vi "Funct img modulation core.vi"(8 "Pockels stay ON for at least this number of us after dwell time":dbl, 9 "Pockels turn ON at least this number of us before fill time completion":dbl, 11 "ROI setup":T1[](array[typedef]) {"ROI group ID" format="%#_6f"; "Laser Power (%)" format="%#_6f"; "Zoom" format="%#_6f"; "Frame Size" format="%#_6f"; "Number of lines" format="%#_6f"; "Composite ID" format="%#_6f"; "Angle (deg)" format="%#_6f"; "ROI Time (ns)" format="%#_6f"; "ROI ID" format="%#_6f"; "Pixels in ROI" format="%#_6f"; "ROI index" format="%#_6f"; "Z stop" format="%#_6f"; "Y stop" format="%#_6f"; "X stop" format="%#_6f"; "Z start" format="%#_6f"; "X start" format="%#_6f"; "Y start" format="%#_6f"}) -> (1 "AO card sampling interval (us)":dbl=1.0 format="%#_13g us", 2 "Fill time (us)":dbl=24.4 format="%#_g us", 3 "waveform out":waveform(dbl), 5 "ROI Dwell Time (us)":dbl)   [LabVIEW 2013]
uses:
  User Interface/Visualisation/Functional Imaging Viewer/Typedefs/ROI parameters data type.ctl
  Typedefs/Rounding type.ctl
  Global Variables/General Globals.vi
  Globals/gl_Pockels control globals.vi
  <vilib>/Waveform/WDTOps.llb/WDT Append Waveforms DBL.vi
panel:
  in  "Disable modulation":bool
  out "Pockels modulation signal":waveform(dbl)(graph)
  out "Remainder (us)":dbl
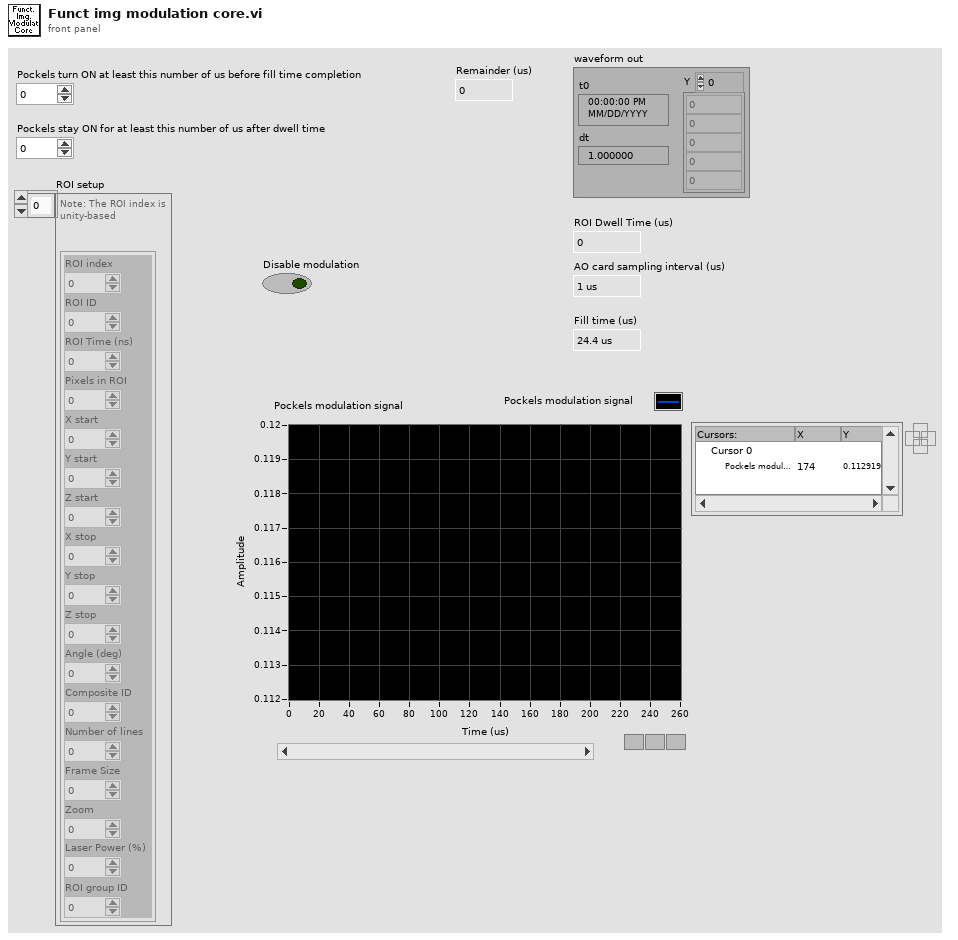
[diagram p1: front panel]
types:
  T1 = typedef "ROI parameters data type.ctl" = cluster{"ROI index":dbl, "ROI ID":dbl, "ROI Time (ns)":dbl, "Pixels in ROI":dbl, "X start":dbl, "Y start":dbl, "Z start":dbl, "X stop":dbl, "Y stop":dbl, "Z stop":dbl, "Angle (deg)":dbl, "Composite ID":dbl, "Number of lines":dbl, "Frame Size":dbl, "Zoom":dbl, "Laser Power (%)":dbl, "ROI group ID":dbl}
  T2 = typedef "Rounding type.ctl" = enum16{"No rounding", "Toward +Inf", "Toward -Inf"}
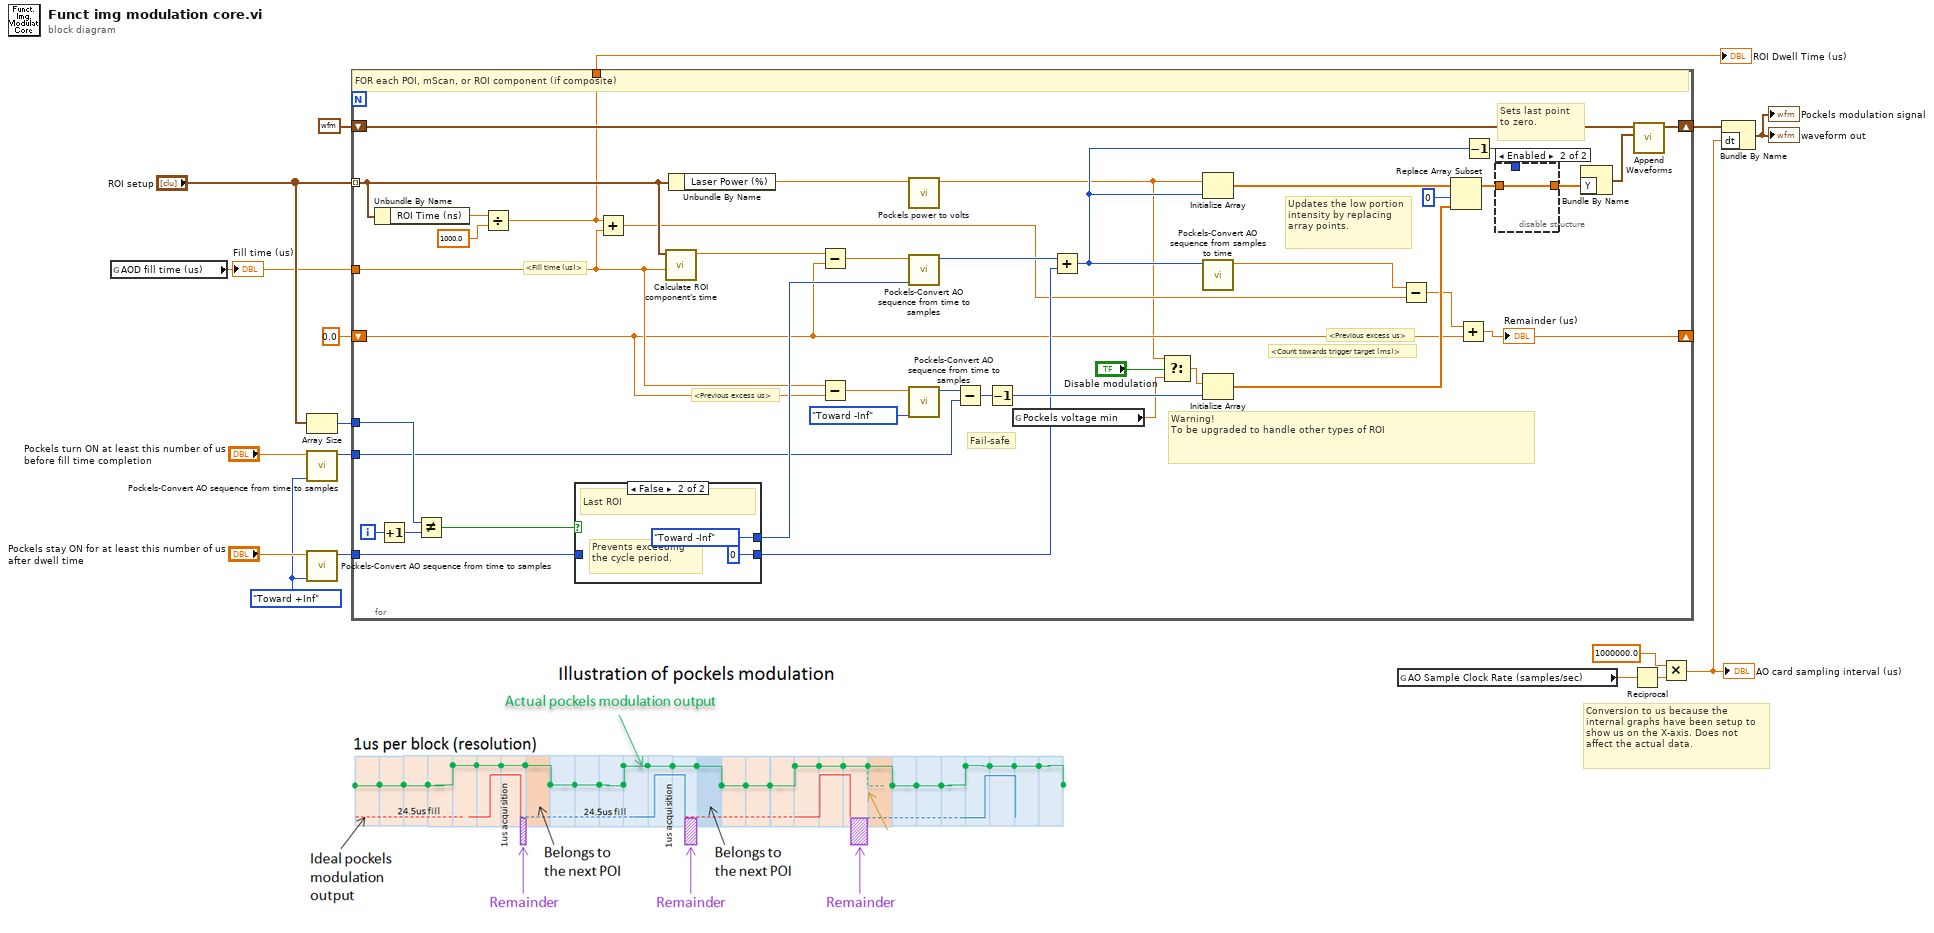
[diagram p0: block diagram]
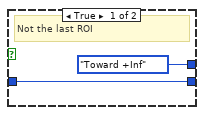
[diagram p2: hidden frame]
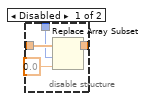
[diagram p3: hidden frame]
diagram:
  w4 = Rounding_type."Toward +Inf" ("Direction (+Inf)")
  # "Conversion to us because the internal graphs have been setup to show us on the X-axis. Does not affect the actual data."
  n1 = global read "General Globals.vi" "AOD fill time (us)"() -> (w8:dbl)
  "Fill time (us)" <- w8
  n2 = Array Size(array="ROI setup") -> (size(s)=w6:i32)
  n3 = call "Pockels-Convert AO sequence from time to samples.vi"("Direction (+Inf)"=w4, "Duration of AO sequence (us)"="Pockels turn ON at least this number of us before fill time completion") -> ("Number of samples in AO sequence"=w5:i32)  [unwired: 9 in]
  n4 = call "Pockels-Convert AO sequence from time to samples.vi"("Direction (+Inf)"=w4, "Duration of AO sequence (us)"="Pockels stay ON for at least this number of us after dwell time") -> ("Number of samples in AO sequence"=w3:i32)  [unwired: 9 in]
  n5 = for {
    tunnel: "ROI setup" -> [w50] mode=indexing
    shift-right: [w45] -> w13
    shift-left: waveform(dbl) {"t0"=timestamp(0 s since 1904-01-01), "dt"=0.0, "Y"=[]} ("waveform out") -> [w55]
    tunnel: w3 -> [w33]
    tunnel: w5 -> [w27]
    shift-right: [w19] -> _
    shift-left: 0.0 ("Count towards trigger target (us)") -> [w28]
    tunnel: w6 -> [w37]
    tunnel: [w35] -> w17
    tunnel: w8 -> [w29]
    i -> [w39]
    # "Updates the low portion intensity by replacing array points."
    # "<Previous excess us>"
    # "<Fill time (us)>"
    # "Warning!\nTo be upgraded to handle other types of ROI"
    # "<Previous excess us>"
    # "<Count towards trigger target (ms)>"
    # "Fail-safe"
    # "Sets last point to zero."
    # "FOR each POI, mScan, or ROI component (if composite)"
    n6 = Unbundle By Name(w50) -> ("ROI Time (ns)"=w36:dbl)
    n7 = Increment(x=w39) -> (x+1=w38:i32)
    n8 = Not Equal?(x=w37, y=w38) -> (x != y?=w24:bool)
    n9 = Divide(x=w36, y=1000.0) -> (x/y=w35:dbl)
    n10 = case shown="False" w24 {
      tunnel: [Rounding_type."Toward +Inf" ("Direction (+Inf)") Rounding_type."Toward -Inf" ("Direction (+Inf)")] -> w31
      tunnel: w33 -> [w60 _]
      tunnel: [w60 0 ("f")] -> w32
      frame True {
        # "Not the last ROI"
      }
      frame False {
        # "Prevents exceeding the cycle period."
        # "Last ROI"
      }
    }
    n11 = Add(x=w35, y=w29) -> (x+y=w26:dbl)
    n12 = call "Calculate ROI component's time.vi"("AOD fill time (us)"=w29, "Normalised ROI setup"=w50) -> ("ROI component's time (us)"=w48:dbl)  [unwired: 9 in]
    n13 = Unbundle By Name(w50) -> ("Laser Power (%)"=w58:dbl)
    n14 = Subtract(x=w48, y=w28) -> (x-y=w47:dbl)
    n15 = Subtract(x=w29, y=w28) -> (x-y=w46:dbl)
    n16 = call "Pockels power to volts.vi"("Pockels power (%)"=w58) -> ("Pockels control voltage (V)"=w21:dbl)  [unwired: 8 in, 2 out]
    n17 = call "Pockels-Convert AO sequence from time to samples.vi"("Direction (+Inf)"=w31, "Duration of AO sequence (us)"=w47) -> ("Number of samples in AO sequence"=w54:i32)  [unwired: 9 in]
    n18 = call "Pockels-Convert AO sequence from time to samples.vi"("Direction (+Inf)"=Rounding_type."Toward -Inf", "Duration of AO sequence (us)"=w46) -> ("Number of samples in AO sequence"=w53:i32)  [unwired: 9 in]
    n19 = Subtract(x=w53, y=w27) -> (x-y=w52:i32)
    n20 = Decrement(x=w52) -> (x-1=w51:i32)
    n21 = global read "gl_Pockels control globals.vi" "Pockels voltage min"() -> (w23:dbl)
    n22 = Add(x=w54, y=w32) -> (x+y=w34:i32)
    n23 = Select(t=w21, s="Disable modulation", f=w23) -> (s? t:f=w22:dbl)
    n24 = Initialize Array(w21, w34) -> (w41:dbl[])
    n25 = call "Pockels-Convert AO sequence from samples to time.vi"("Number of samples in AO sequence"=w34) -> ("Duration of AO sequence (us)"=w25:dbl)  [unwired: 10 in]
    n26 = Initialize Array(w22, w51) -> (w57:dbl[])
    n27 = Subtract(x=w25, y=w26) -> (x-y=w43:dbl)
    n28 = Replace Array Subset(array=w41, new element=w57, index=0) -> (w42:dbl[])
    n29 = Add(x=w43, y=w28) -> (x+y=w19:dbl)
    "Remainder (us)" <- w19
    n30 = Decrement(x=w34) -> (x-1=w40:i32)
    n31 = disable-structure shown="Enabled" {
      disable-tunnel: w42 -> [w66 w67]
      disable-tunnel: [w65 w67] -> w18
      disable-tunnel: w40 -> [w63 _]
      frame Disabled {
        n32 = Replace Array Subset(array=w66, new element=0.0 ("new element/subarray"), index=w63) -> (w65:dbl[])
      }
      frame Enabled {
      }
    }
    n33 = Bundle By Name("Y"=w18) -> (w44:waveform(dbl))  [unwired: 1 in]
    n34 = call-poly <vilib>:"Append Waveforms.vi"("waveform B"=w44, "waveform A"=w55) -> ("waveform out"=w45:waveform(dbl))  [unwired: 8 in, 1 out]
  }
  "ROI Dwell Time (us)" <- w17
  n35 = global read "General Globals.vi" "AO Sample Clock Rate (samples/sec)"() -> (w14:dbl)
  n36 = Reciprocal(x=w14) -> (1/x=w15:dbl)
  n37 = Multiply(x=1000000.0, y=w15) -> (x*y=w12:dbl)
  "AO card sampling interval (us)" <- w12
  n38 = Bundle By Name(cluster=w13, "dt"=w12) -> (→"waveform out" →"Pockels modulation signal":waveform(dbl))
